vi "serial open.vi"(8 "error in (no error)":errorcluster, 11 "port":string="/dev/ttyACM0") -> (0 "error out":errorcluster, 3 "portHandle":i32)   [LabVIEW 2025]
uses:
  libc.so.6
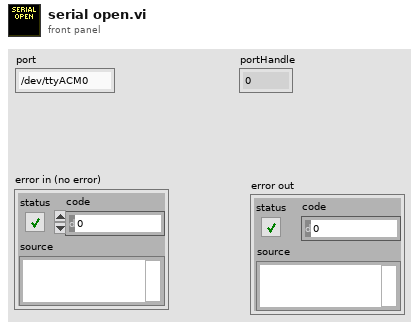
[diagram p1: front panel]
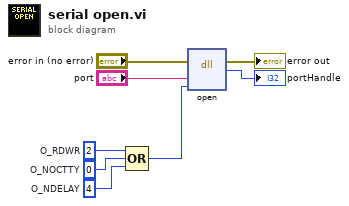
[diagram p0: block diagram]
diagram:
  w2 = u16 4  # O_NDELAY
  w3 = u16 0  # O_NOCTTY
  w4 = u16 2  # O_RDWR
  n1 = Compound Arithmetic op=OR(w4, w3, w2) -> (w1:u16)
  n2 = dll-call lib="libc.so.6" fn="open"(error in="error in (no error)", "portName"="port", "mode"=w1) -> (error out=→"error out":errorcluster, "return type"=→"portHandle":i32)  [unwired: 4 in, 1 out]
